vi "02 Triple Waveform Simulation (x64-2018).vi"() -> ()   [LabVIEW 2017]
panel:
  in  "DAQmx Task Name":refnum<k21>
  out "Waveform Graph":waveform(dbl)[](graph)
  out "error out":errorcluster
  in  "Samples per Channel":dbl(slide) scale=1.0..200.0
  in  "Rate":dbl(slide)=5.0 scale=5.0..2000.0
  in  "stop":bool
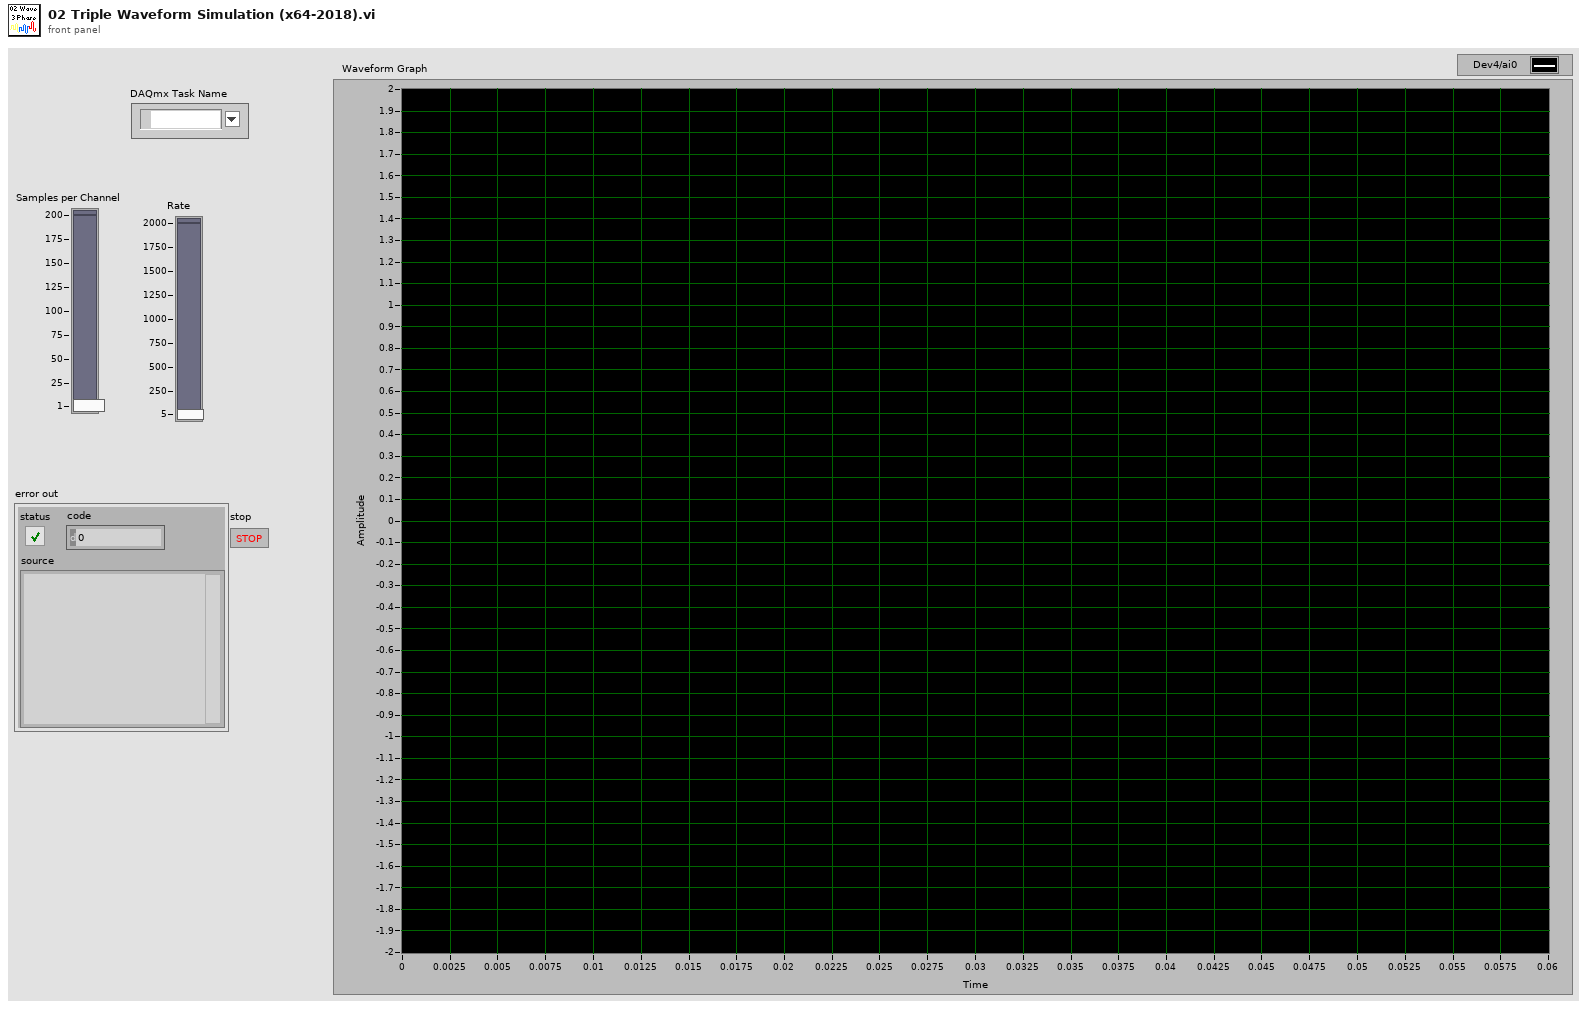
[diagram p1: front panel]
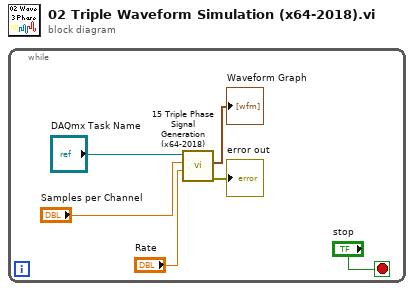
[diagram p0: block diagram]
diagram:
  n1 = while {
    stop <- "stop" stop-if-true
    n2 = call "15 Triple Phase Signal Generation (x64-2018).vi"("Rate"="Rate", "Number of samples per channel"="Samples per Channel", "task/channels in"="DAQmx Task Name") -> ("Error Out"=→"error out":errorcluster, "data"=→"Waveform Graph":waveform(dbl)[])  [unwired: 6 in, 1 out]
  }
